vi "ResponseValue.vi"(0 "StepMotor in":refnum<class "StepMotor.lvclass">, 11 "error in (no error)":errorcluster) -> (4 "StepMotor out":refnum<class "StepMotor.lvclass">, 15 "error out":errorcluster)   [LabVIEW 2010, in "StepMotor.lvclass"]
doc: "Декодирование прочитанного сообщения и разбиение выделение из сообщения значения параметра."
uses:
  StepMotor.lvclass
  StepMotor.lvclass/StepMotor.ctl
panel:
  in  "Количество бит":u16(ring) items=["4", "4", "2", "2", "2", "2", "2", "2", "4", "4", "4", "4", "4", "4", "4", "4", "2", "4", "2", "2", "4", "2", "2", "2", "2", "2", "2", "2", "4", "4", "4", "4", "4", "4", "4", "4", "4", "4", "4", "4", "2", "2", "4", "4", "4", "4", "4", "4", "2", "2", "2", "2", "2", "2", "2", "2", "2", "2", "2", "2", "2", "2", "2", "2", "2", "2", "2", "2", "2", "4", "4", "2", "2", "2", "2", "2", "1", "2", "2", "4", "4", "4", "2", "2", "2", "2", "2", "2", "4", "4", "2", "2", "2", "2", "2", "2", "4", "2", "2", "2", "4", "2", "4", "4", "4", "4", "4", "4", "2", "2", "2", "2", "4", "2", "4", "4", "2", "4", "2", "2", "4", "2", "2", "2", "2", "4", "2", "2", "2", "2", "2", "2", "2", "2", "2", "2", "2", "4", "4", "2", "2", "2", "2", "4", "4", "2", "2", "2", "2", "2", "2", "2", "4", "4", "4", "4", "4", "4", "4", "4", "4", "4", "4", "4", "4", "4", "4", "4", "2", "4", "4", "4", "4", "4", "4", "4", "4", "2", "2", "2", "2", "2", "2", "2", "2", "2", "2", "2", "2", "2", "2", "4", "4", "4", "4", "4", "4", "4", "4", "4", "4", "4", "4", "4", "4", "4", "4", "4", "4", "4", "4"]
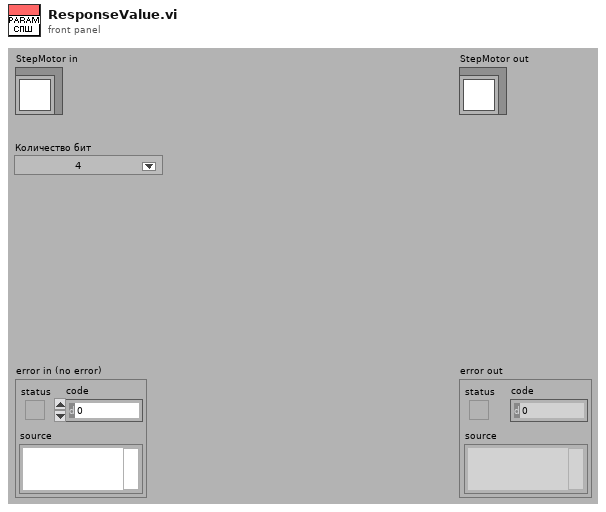
[diagram p1: front panel]
types:
  T1 = enum32{"cp1", "cp2", "cp3", "cp4", "cp5", "cp6", "cp7", "cp8", "cp9", "cp10", "cp11", "cp12", "vp1", "vp2", "vp16", "vp3", "vp4", "vp5", "vp6", "vp7", "vp8", "vp9", "vp10", "vp11", "vp12", "vp13", "vp14", "vp15", "vp17", "vp18", "vp19", "vp20", "vp21", "vp22", "vp23", "vp24", "vp25", "vp26", "pp1", "pp2", "pp3", "pp5", "pp6", "pp7", "pp8", "pp9", "pp10", "pp11", "ss1", "ss2", "ss3", "ss4", "ss5", "ss6", "ss7", "ss8", "ss9", "ss10", "ss11", "ss12", "ss13", "ss14", "ss15", "si1", "si2", "ss16", "ss17", "ss18", "ct1", "ct2", "ct3", "dd1", "dd6", "dd3", "dd9", "dd2", "dd4", "dd5", "dd21", "dd7", "dd8", "dd20", "dd10", "dd19", "dd12", "dd11", "dd13", "dd14", "dd15", "dd16", "dd17", "dd18", "dd22", "dd23", "dd24", "dd25", "dd26", "dd27", "dd28", "dd29", "dd30", "dd31", "dd32", "dd33", "dd34", "st1", "st2", "st3", "st4", "st5", "st6", "st7", "st8", "st9", "st10", "st11", "st12", "st13", "st14", "tp1", "tp3", "tp2", "tp5", "tp6", "ip0", "ip1", "ip2", "ip3", "ip4", "ip5", "ip6", "ip7", "ip8", "ip9", "ip10", "ip11", "ip12", "ip13", "ip14", "ip15", "ip16", "ip17", "ip18", "ip19", "ip20", "ep1", "ep2", "ep3", "ep4", "ep5", "ep6", "ep7", "up0", "up1", "up2", "up3", "up4", "up5", "up6", "up7", "up8", "up9", "up10", "up11", "up12", "up13", "up14", "up15", "up16", "up17", "up18", "up19", "up20", "up21", "up22", "up23", "up24", "io0", "io1", "io2", "io3", "io4", "io5", "io6", "io7", "io8", "io9", "io10", "io11", "io12", "io13", "io14", "pd1", "pd2", "pd3", "pd4", "pd5", "pd6", "pd7", "pd8", "pd9", "pd10", "pd11", "pd12", "pd13", "pd14", "pd15", "pd16", "pd17", "pd18", "pd19", " "}
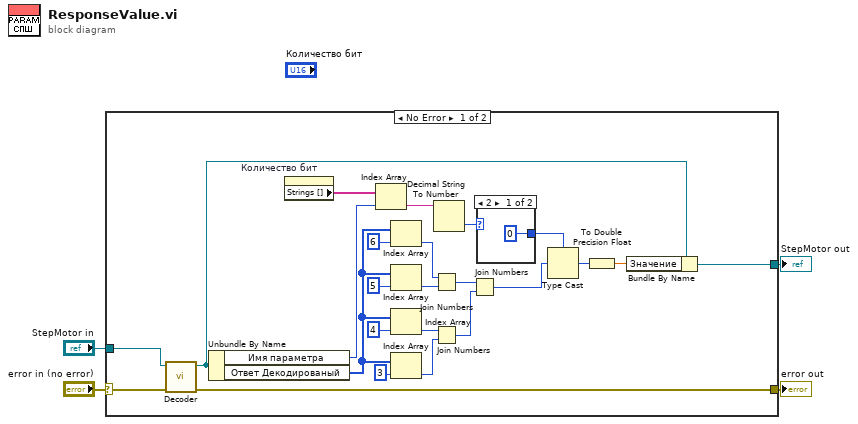
[diagram p0: block diagram]
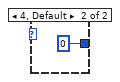
[diagram p2: hidden frame]
diagram:
  n1 = case shown="No Error" "error in (no error)" {
    selector: "error in (no error)" -> [w28 w32]
    tunnel: [w22 w32] -> w3
    tunnel: [w21 w31] -> w1
    tunnel: "StepMotor in" -> [w27 w31]
    frame No Error {
      n2 = call "Decoder.vi"("error in (no error)"=w28, "StepMotor in"=w27) -> ("error out"=w22:errorcluster, "StepMotor out"=w23:refnum<class "StepMotor.lvclass">)  [unwired: 8 in]
      n3 = Unbundle By Name(w23) -> ("Имя параметра"=w19:T1, "Ответ Декодированый"=w13:u8[])
      n4 = property on="Количество бит" class="Ring (strict)"() -> ("Strings []"=w20:string[])  [unwired: 2 in, 2 out]
      n5 = Index Array(array=w20, index=w19) -> (element=w14:string)
      n6 = Index Array(array=w13, index=6) -> (element=w11:u8)
      n7 = Index Array(array=w13, index=5) -> (element=w10:u8)
      n8 = Index Array(array=w13, index=4) -> (element=w9:u8)
      n9 = Index Array(array=w13, index=3) -> (element=w8:u8)
      n10 = Join Numbers(hi=w11, lo=w10) -> ((hi.lo)=w6:u16)
      n11 = Join Numbers(hi=w9, lo=w8) -> ((hi.lo)=w7:u16)
      n12 = Decimal String To Number(string=w14) -> (number=w12:i32)  [unwired: 2 in, 1 out]
      n13 = Join Numbers(hi=w6, lo=w7) -> ((hi.lo)=w16:u32)
      n14 = case shown="2" w12 {
        tunnel: [i16 0 ("Значение") 0 ("Значение")] -> w5
        frame 2 {
        }
        frame 4, Default {
        }
      }
      n15 = Type Cast(type=w5, x=w16) -> (*(type *) &x=w18:i32)
      n16 = To Double Precision Float(number=w18) -> (double precision float=w17:dbl)
      n17 = Bundle By Name(cluster=w23, "Значение"=w17) -> (w21:refnum<class "StepMotor.lvclass">)
    }
    frame Error {
    }
  }
  "error out" <- w3
  "StepMotor out" <- w1
